vi "Temperature_UDC.vi"(2 "Debug Mode":bool, 3 "Elapsed Time (s)":dbl, 4 "State":enum16{"Edit", "Start", "Run", "End", "Idle"}(ring), 5 "Argument List In":string[](array[string])) -> (0 "Status Out":string, 1 "Argument List Out":string[](array[string]))   [LabVIEW 2011]
panel:
  in  "Cancel":bool
  in  "OK":bool
  out "Temperature":dbl
  out "Read Cycle":dbl
  out "Timer":dbl
  out "Previous Time":dbl
  in  "Setpoint (C)":dbl
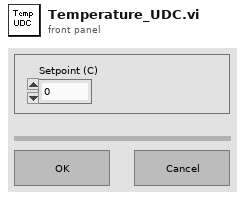
[diagram p1: front panel]
types:
  T1 = enum16{"Discrete", "Continuous", "Instantaneous"}
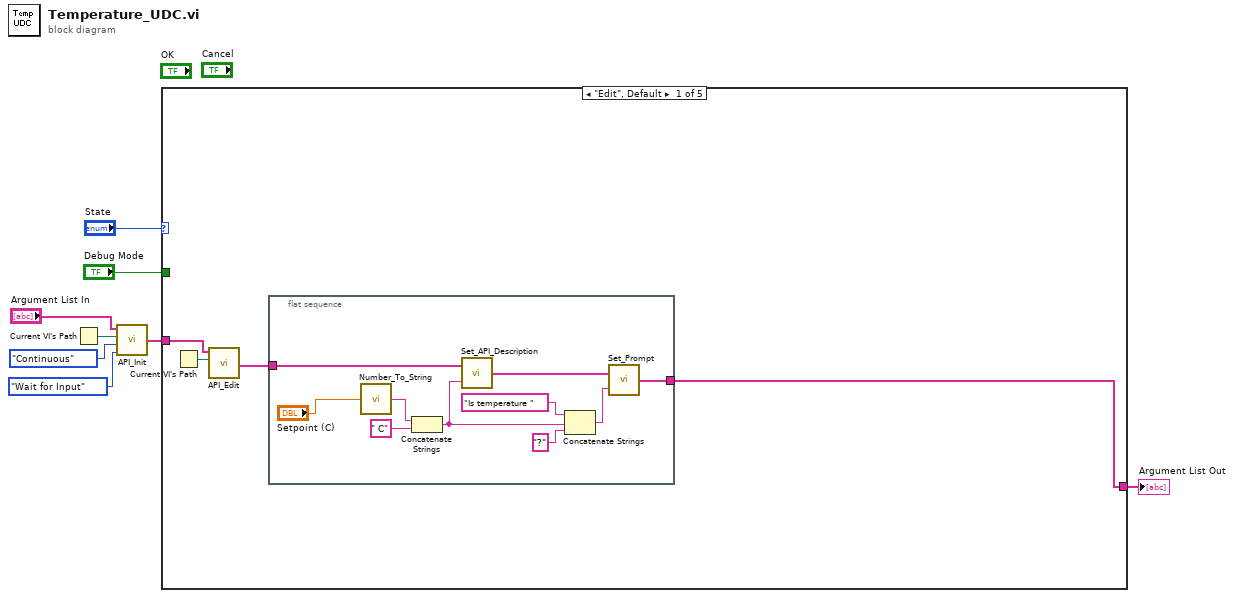
[diagram p0: block diagram]
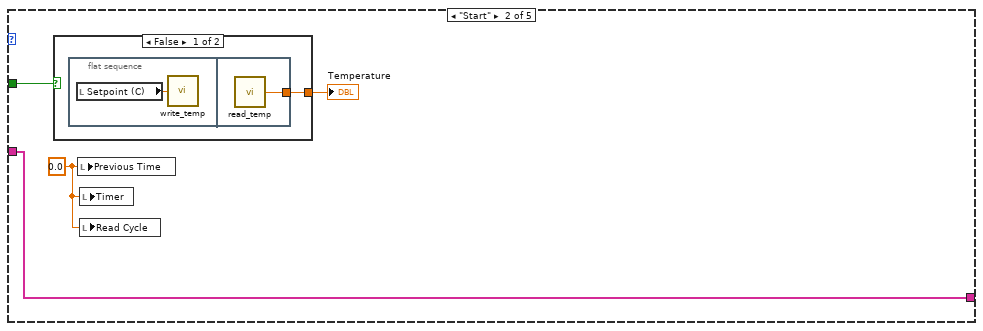
[diagram p2: hidden frame]
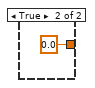
[diagram p3: hidden frame]
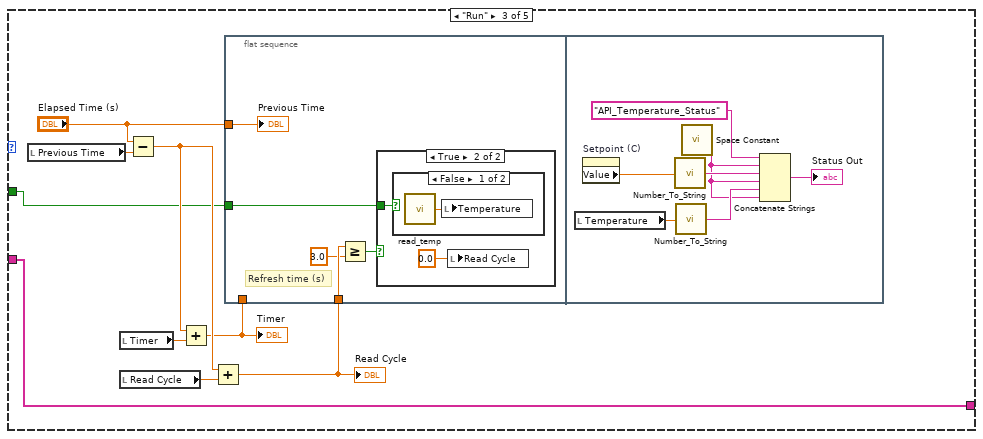
[diagram p4: hidden frame]
diagram:
  n1 = Current VI's Path() -> (path=w5:path)
  n2 = call "API_Init.vi"("API Option"=enum16{"None", "Blocking", "Wait for Input"}."Wait for Input", "API Mode"=T1."Continuous", "VI Path"=w5, "Argument List In"="Argument List In") -> ("Argument List Out"=w2:string[])
  n3 = case shown="\"Edit\", Default" "State" {
    tunnel: [w9 w26 w39 w55 w56] -> w7
    tunnel: w2 -> [w11 w26 w39 w55 w56]
    tunnel: "Debug Mode" -> [_ w25 w31 _ _]
    frame "Edit", Default {
      n4 = Current VI's Path() -> (path=w12:path)
      n5 = call "API_Edit.vi"("VI Path"=w12, "Argument List In"=w11) -> ("Argument List Out"=w10:string[])  [unwired: 2 in]
      n6 = flat-sequence {
        tunnel: w10 -> [w16]
        tunnel: [w14] -> w9
        frame #0 {
          n7 = call "Number_To_String.vi"("Number"="Setpoint (C)") -> ("String"=w15:string)
          n8 = Concatenate Strings(w15, " C" ("string")) -> (w20:string)
          n9 = call "Set_API_Description.vi"("Description"=w20, "Argument List In"=w16) -> ("Argument List Out"=w21:string[])
          n10 = Concatenate Strings("Is temperature " ("Prompt"), w20, "?" ("string")) -> (w17:string)
          n11 = call "Set_Prompt.vi"("Prompt"=w17, "Argument List In"=w21) -> ("Argument List Out"=w14:string[])
        }
      }
    }
    frame "Start" {
      w24 = 0.0 ("Previous Time")
      n12 = case shown="False" w25 {
        tunnel: [w27 0.0 ("Temperature (C)")] -> w23
        frame False {
          n13 = flat-sequence {
            tunnel: [w29] -> w27
            frame #0 {
              n14 = local read "Setpoint (C)"() -> (w28:dbl)
              n15 = call "write_temp.vi"("Temperature (C)"=w28) -> ()  [unwired: 1 out]
            }
            frame #1 {
              n16 = call "read_temp.vi"() -> ("Temperature (C)"=w29:dbl)  [unwired: 1 out]
            }
          }
        }
        frame True {
        }
      }
      "Temperature" <- w23
      n17 = local write "Previous Time"(w24) -> ()
      n18 = local write "Timer"(w24) -> ()
      n19 = local write "Read Cycle"(w24) -> ()
    }
    frame "Run" {
      n20 = local read "Previous Time"() -> (w37:dbl)
      n21 = local read "Timer"() -> (w36:dbl)
      n22 = local read "Read Cycle"() -> (w35:dbl)
      n23 = Subtract(x="Elapsed Time (s)", y=w37) -> (x-y=w34:dbl)
      n24 = Add(x=w34, y=w36) -> (x+y=w32:dbl)
      "Timer" <- w32
      n25 = Add(x=w34, y=w35) -> (x+y=w33:dbl)
      "Read Cycle" <- w33
      n26 = flat-sequence {
        tunnel: w32 -> [_]
        tunnel: w33 -> [w43]
        tunnel: "Elapsed Time (s)" -> [w44]
        tunnel: w31 -> [w40]
        frame #0 {
          # "Refresh time (s)"
          n27 = Greater Or Equal?(x=w43, y=3.0) -> (x >= y?=w41:bool)
          n28 = case shown="True" w41 {
            tunnel: w40 -> [_ w45]
            frame False {
            }
            frame True {
              n29 = case shown="False" w45 {
                frame False {
                  n30 = call "read_temp.vi"() -> ("Temperature (C)"=w47:dbl)  [unwired: 1 out]
                  n31 = local write "Temperature"(w47) -> ()
                }
                frame True {
                }
              }
              n32 = local write "Read Cycle"(0.0 ("Read Cycle")) -> ()
            }
          }
          "Previous Time" <- w44
        }
        frame #1 {
          n33 = local read "Temperature"() -> (w48:dbl)
          n34 = property on="Setpoint (C)" class="DigNum (strict)"() -> ("Value"=w50:dbl)  [unwired: 2 in, 2 out]
          n35 = call "Number_To_String.vi"("Number"=w50) -> ("String"=w54:string)
          n36 = call "Number_To_String.vi"("Number"=w48) -> ("String"=w53:string)
          n37 = call <vilib>:"Space Constant.vi"() -> ("String"=w51:string)
          n38 = Concatenate Strings("API_Temperature_Status" ("string"), w51, w54, w51, w53, w51) -> (→"Status Out":string)
        }
      }
    }
    frame "End" {
    }
    frame "Idle" {
    }
  }
  "Argument List Out" <- w7
